vi "Find_Binary_Wavedump.vi"(8 "Time Limit (s)":u32) -> (12 "File Not Found":bool, 13 "File Not Found 5":bool, 14 "File Not Found 2":bool, 15 "File Not Found 6":bool, 16 "File Not Found 3":bool, 17 "File Not Found 7":bool, 18 "File Not Found 4":bool, 19 "File Not Found 8":bool, 20 "File Found":bool, 21 "File Found 2":bool, 22 "File Found 3":bool, 23 "File Found 4":bool, 24 "File Found 5":bool, 25 "File Found 6":bool, 26 "File Found 7":bool, 27 "File Found 8":bool)   [LabVIEW 2018]
panel:
  in  "Channel":string[](array[string])
  in  "Test":string(combo)
  out "File Found":bool[](array[boolean])
  out "File Not Found":bool[](array[boolean])
  out "File Path Out 8":path
  out "Time Looking for File (s) 8":u32=17125
  out "File Path Out 7":path
  out "Time Looking for File (s) 7":u32=17125
  out "File Path Out 6":path
  out "Time Looking for File (s) 6":u32=17125
  out "File Path Out 5":path
  out "Time Looking for File (s) 5":u32=17125
  out "File Path Out 4":path
  out "Time Looking for File (s) 4":u32=17125
  out "File Path Out 3":path
  out "Time Looking for File (s) 3":u32=17125
  out "File Path Out 2":path
  out "Time Looking for File (s) 2":u32=17125
  out "File Path Out":path
  out "Time Looking for File (s)":u32=17125
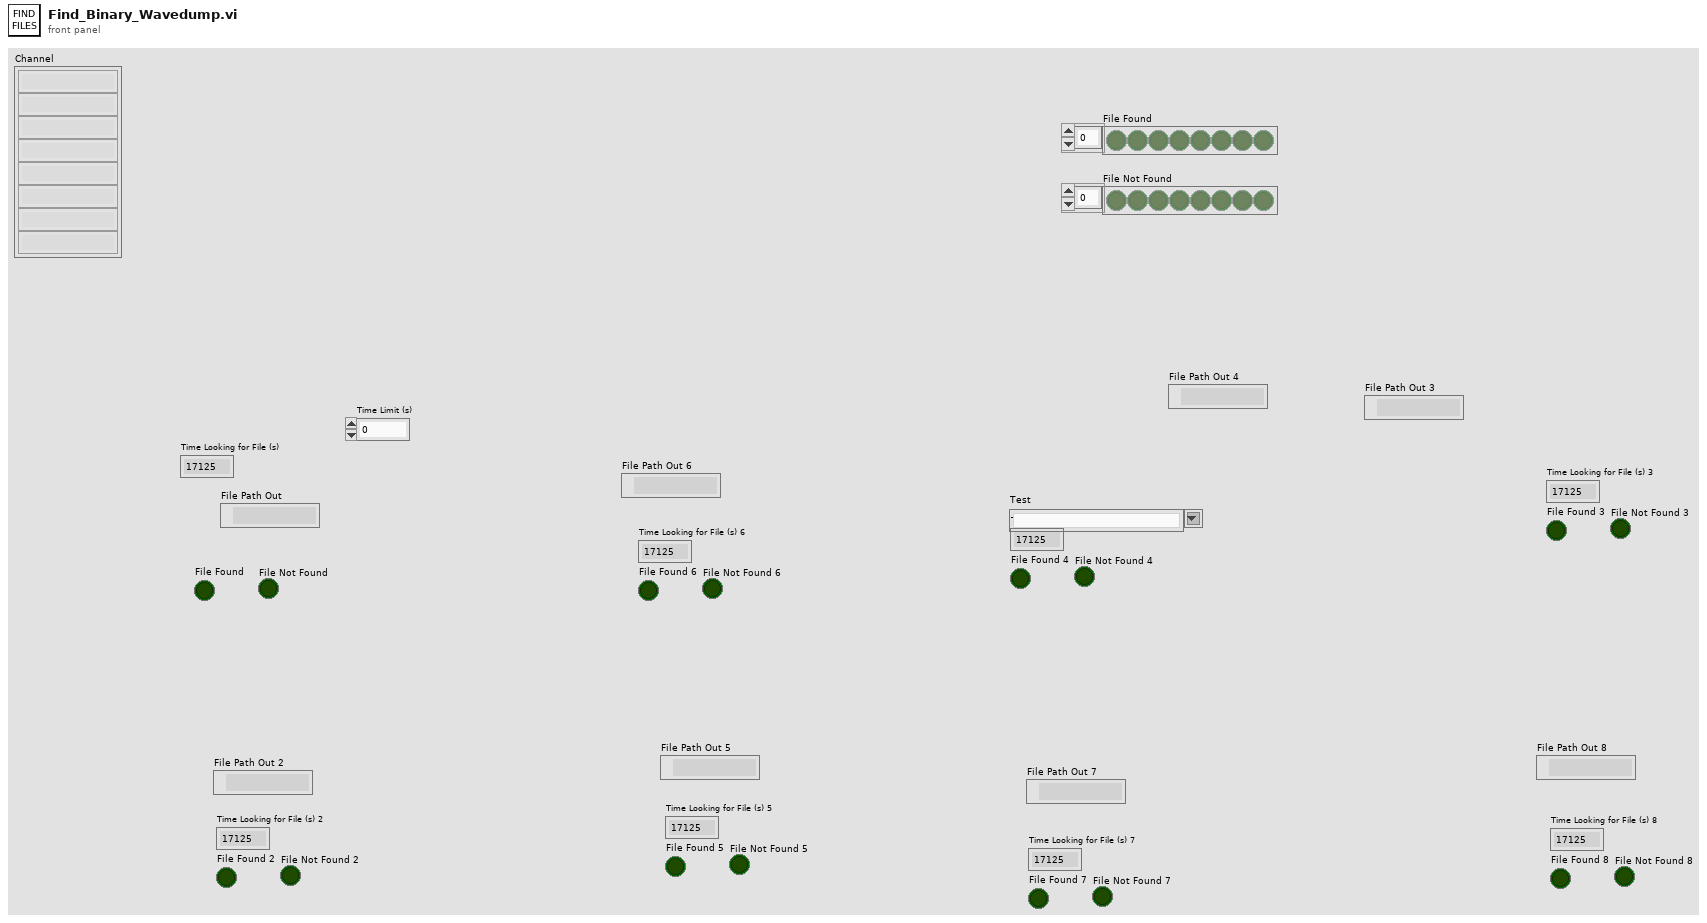
[diagram p1: front panel]
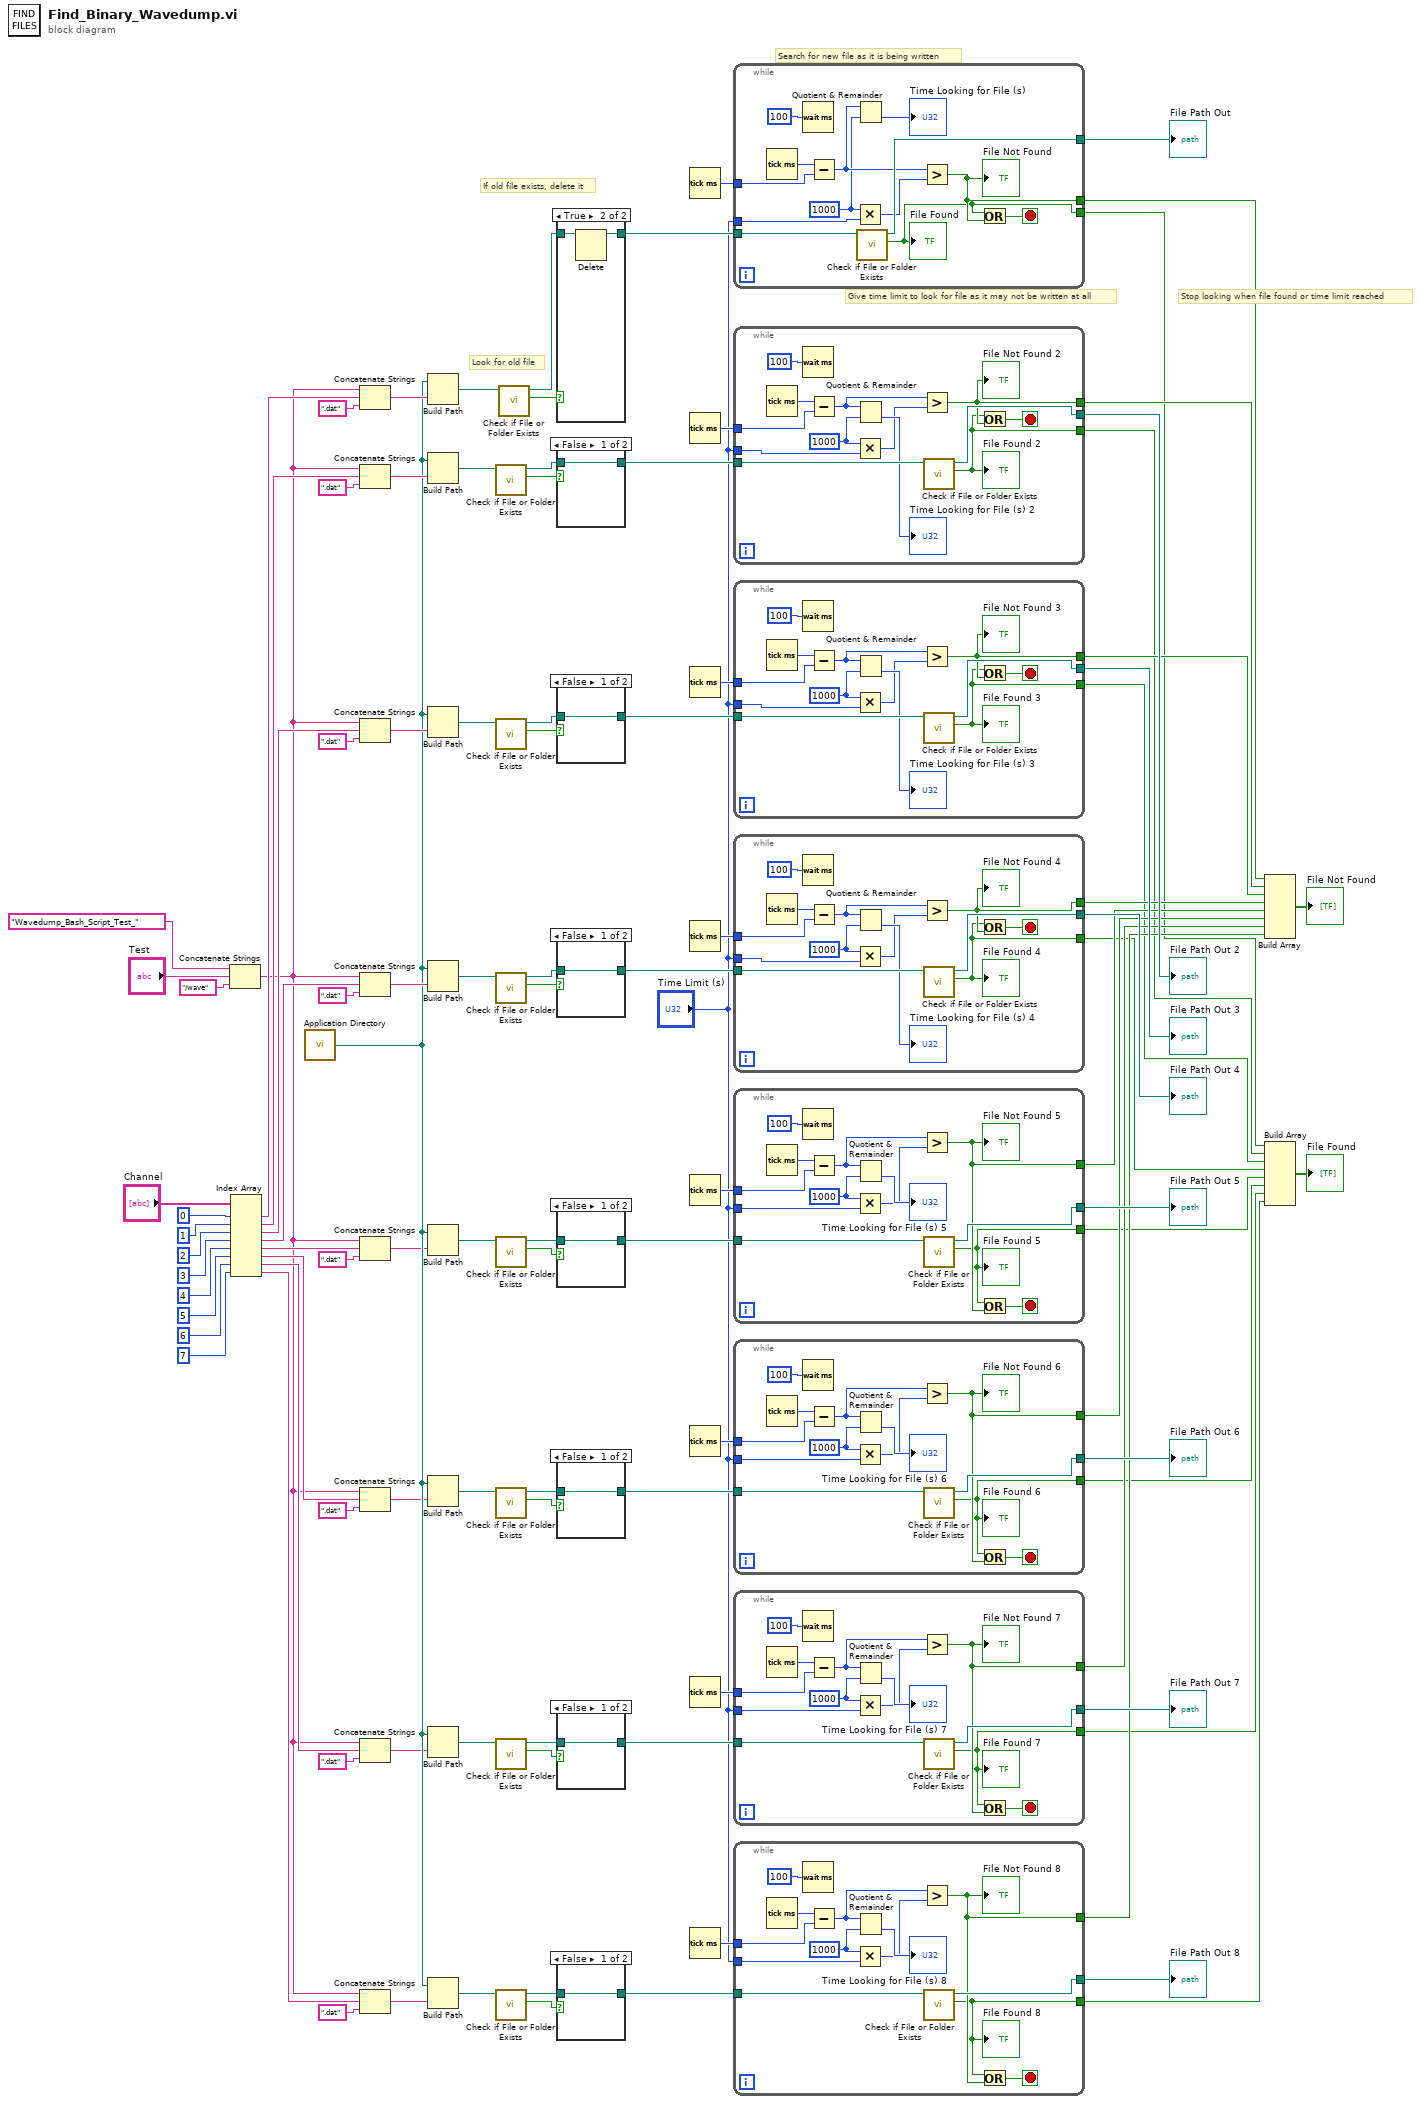
[diagram p0: block diagram]
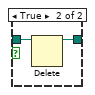
[diagram p2: hidden frame]
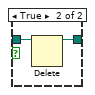
[diagram p3: hidden frame]
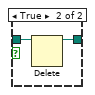
[diagram p4: hidden frame]
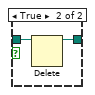
[diagram p5: hidden frame]
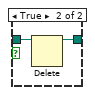
[diagram p6: hidden frame]
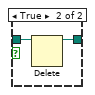
[diagram p7: hidden frame]
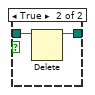
[diagram p8: hidden frame]
diagram:
  # "Stop looking when file found or time limit reached"
  # "Give time limit to look for file as it may not be written at all"
  # "Search for new file as it is being written"
  # "Look for old file"
  # "If old file exists, delete it"
  n1 = Concatenate Strings("Wavedump_Bash_Script_Test_" ("string"), "Test", "/wave" ("string")) -> (w16:string)
  n2 = Index Array(array="Channel", index #1=0 ("index"), index #2=1 ("index"), index #3=2 ("index"), index #4=3 ("index"), index #5=4 ("index"), index #6=5 ("index"), index #7=6 ("index"), index #8=7 ("index")) -> (element #1=w31:string, element #2=w23:string, element #3=w22:string, element #4=w21:string, element #5=w20:string, element #6=w19:string, element #7=w18:string, element #8=w17:string)
  n3 = call <vilib>:"Application Directory.vi"() -> ("Application Directory"=w11:path)
  n4 = Concatenate Strings(w16, w31, ".dat" ("string")) -> (w42:string)
  n5 = Concatenate Strings(w16, w23, ".dat" ("string")) -> (w14:string)
  n6 = Concatenate Strings(w16, w22, ".dat" ("string")) -> (w15:string)
  n7 = Concatenate Strings(w16, w21, ".dat" ("string")) -> (w13:string)
  n8 = Concatenate Strings(w16, w20, ".dat" ("string")) -> (w10:string)
  n9 = Concatenate Strings(w16, w19, ".dat" ("string")) -> (w9:string)
  n10 = Concatenate Strings(w16, w18, ".dat" ("string")) -> (w8:string)
  n11 = Concatenate Strings(w16, w17, ".dat" ("string")) -> (w7:string)
  n12 = Build Path(base path=w11, name or relative path=w42) -> (appended path=w30:path)
  n13 = Build Path(base path=w11, name or relative path=w14) -> (appended path=w12:path)
  n14 = Build Path(base path=w11, name or relative path=w15) -> (appended path=w6:path)
  n15 = Build Path(base path=w11, name or relative path=w13) -> (appended path=w5:path)
  n16 = Build Path(base path=w11, name or relative path=w10) -> (appended path=w4:path)
  n17 = Build Path(base path=w11, name or relative path=w9) -> (appended path=w1:path)
  n18 = Build Path(base path=w11, name or relative path=w8) -> (appended path=w3:path)
  n19 = Build Path(base path=w11, name or relative path=w7) -> (appended path=w2:path)
  n20 = call <vilib>:"Check if File or Folder Exists.vi"("path"=w12) -> ("file or folder exists?"=w99:bool, "dup path"=w100:path)  [unwired: 8 in, 1 out]
  n21 = call <vilib>:"Check if File or Folder Exists.vi"("path"=w6) -> ("file or folder exists?"=w94:bool, "dup path"=w95:path)  [unwired: 8 in, 1 out]
  n22 = call <vilib>:"Check if File or Folder Exists.vi"("path"=w5) -> ("file or folder exists?"=w89:bool, "dup path"=w90:path)  [unwired: 8 in, 1 out]
  n23 = call <vilib>:"Check if File or Folder Exists.vi"("path"=w4) -> ("file or folder exists?"=w84:bool, "dup path"=w85:path)  [unwired: 8 in, 1 out]
  n24 = call <vilib>:"Check if File or Folder Exists.vi"("path"=w1) -> ("file or folder exists?"=w79:bool, "dup path"=w80:path)  [unwired: 8 in, 1 out]
  n25 = call <vilib>:"Check if File or Folder Exists.vi"("path"=w3) -> ("file or folder exists?"=w74:bool, "dup path"=w75:path)  [unwired: 8 in, 1 out]
  n26 = call <vilib>:"Check if File or Folder Exists.vi"("path"=w2) -> ("file or folder exists?"=w69:bool, "dup path"=w70:path)  [unwired: 8 in, 1 out]
  n27 = call <vilib>:"Check if File or Folder Exists.vi"("path"=w30) -> ("file or folder exists?"=w104:bool, "dup path"=w105:path)  [unwired: 8 in, 1 out]
  n28 = case shown="True" w104 {
    tunnel: w105 -> [w106 w108]
    tunnel: [w106 w107] -> w103
    frame False {
    }
    frame True {
      n29 = Delete(path (use dialog)=w108) -> (deleted path=w107:path)  [unwired: 4 in, 2 out]
    }
  }
  n30 = case shown="False" w99 {
    tunnel: w100 -> [w109 w111]
    tunnel: [w109 w110] -> w98
    frame False {
    }
    frame True {
      n31 = Delete(path (use dialog)=w111) -> (deleted path=w110:path)  [unwired: 4 in, 2 out]
    }
  }
  n32 = case shown="False" w94 {
    tunnel: w95 -> [w112 w114]
    tunnel: [w112 w113] -> w93
    frame False {
    }
    frame True {
      n33 = Delete(path (use dialog)=w114) -> (deleted path=w113:path)  [unwired: 4 in, 2 out]
    }
  }
  n34 = case shown="False" w89 {
    tunnel: w90 -> [w115 w117]
    tunnel: [w115 w116] -> w88
    frame False {
    }
    frame True {
      n35 = Delete(path (use dialog)=w117) -> (deleted path=w116:path)  [unwired: 4 in, 2 out]
    }
  }
  n36 = case shown="False" w84 {
    tunnel: w85 -> [w118 w120]
    tunnel: [w118 w119] -> w83
    frame False {
    }
    frame True {
      n37 = Delete(path (use dialog)=w120) -> (deleted path=w119:path)  [unwired: 4 in, 2 out]
    }
  }
  n38 = case shown="False" w79 {
    tunnel: w80 -> [w121 w123]
    tunnel: [w121 w122] -> w78
    frame False {
    }
    frame True {
      n39 = Delete(path (use dialog)=w123) -> (deleted path=w122:path)  [unwired: 4 in, 2 out]
    }
  }
  n40 = case shown="False" w74 {
    tunnel: w75 -> [w124 w126]
    tunnel: [w124 w125] -> w73
    frame False {
    }
    frame True {
      n41 = Delete(path (use dialog)=w126) -> (deleted path=w125:path)  [unwired: 4 in, 2 out]
    }
  }
  n42 = case shown="False" w69 {
    tunnel: w70 -> [w127 w129]
    tunnel: [w127 w128] -> w68
    frame False {
    }
    frame True {
      n43 = Delete(path (use dialog)=w129) -> (deleted path=w128:path)  [unwired: 4 in, 2 out]
    }
  }
  n44 = Tick Count (ms)() -> (millisecond timer value=w102:u32)
  n45 = Tick Count (ms)() -> (millisecond timer value=w97:u32)
  n46 = Tick Count (ms)() -> (millisecond timer value=w92:u32)
  n47 = Tick Count (ms)() -> (millisecond timer value=w87:u32)
  n48 = Tick Count (ms)() -> (millisecond timer value=w82:u32)
  n49 = Tick Count (ms)() -> (millisecond timer value=w77:u32)
  n50 = Tick Count (ms)() -> (millisecond timer value=w72:u32)
  n51 = Tick Count (ms)() -> (millisecond timer value=w67:u32)
  n52 = while {
    tunnel: [w142] -> w101
    tunnel: w102 -> [w140]
    tunnel: w103 -> [w138]
    tunnel: [w136] -> w65
    tunnel: "Time Limit (s)" -> [w131]
    tunnel: [w130] -> w48
    stop <- w137 stop-if-true
    w133 = u32 1000 ("y")
    n53 = Tick Count (ms)() -> (millisecond timer value=w139:u32)
    n54 = Wait (ms)(milliseconds to wait=100) -> ()  [unwired: 1 out]
    n55 = Subtract(x=w139, y=w140) -> (x-y=w134:u32)
    n56 = Multiply(x=w133, y=w131) -> (x*y=w132:u32)
    n57 = Quotient & Remainder(x=w134, y=w133) -> (floor(x/y)=→"Time Looking for File (s)":u32)  [unwired: 1 out]
    n58 = call <vilib>:"Check if File or Folder Exists.vi"("path"=w138) -> ("file or folder exists?"=w130:bool, "dup path"=w142:path)  [unwired: 8 in, 1 out]
    "File Found" <- w130
    n59 = Greater?(x=w134, y=w132) -> (0:w136:bool)
    "File Not Found" <- w136
    n60 = Or(x=w130, y=w136) -> (x .or. y?=w137:bool)
  }
  "File Path Out" <- w101
  n61 = while {
    tunnel: [w155] -> w96
    tunnel: w97 -> [w153]
    tunnel: w98 -> [w151]
    tunnel: [w149] -> w64
    tunnel: "Time Limit (s)" -> [w144]
    tunnel: [w143] -> w50
    stop <- w150 stop-if-true
    w146 = u32 1000 ("y")
    n62 = Tick Count (ms)() -> (millisecond timer value=w152:u32)
    n63 = Wait (ms)(milliseconds to wait=100) -> ()  [unwired: 1 out]
    n64 = Subtract(x=w152, y=w153) -> (x-y=w147:u32)
    n65 = Multiply(x=w146, y=w144) -> (x*y=w145:u32)
    n66 = Quotient & Remainder(x=w147, y=w146) -> (floor(x/y)=→"Time Looking for File (s) 2":u32)  [unwired: 1 out]
    n67 = Greater?(x=w147, y=w145) -> (0:w149:bool)
    "File Not Found 2" <- w149
    n68 = call <vilib>:"Check if File or Folder Exists.vi"("path"=w151) -> ("file or folder exists?"=w143:bool, "dup path"=w155:path)  [unwired: 8 in, 1 out]
    "File Found 2" <- w143
    n69 = Or(x=w143, y=w149) -> (x .or. y?=w150:bool)
  }
  "File Path Out 2" <- w96
  n70 = while {
    tunnel: [w168] -> w91
    tunnel: w92 -> [w166]
    tunnel: w93 -> [w164]
    tunnel: [w162] -> w63
    tunnel: "Time Limit (s)" -> [w157]
    tunnel: [w156] -> w49
    stop <- w163 stop-if-true
    w159 = u32 1000 ("y")
    n71 = Tick Count (ms)() -> (millisecond timer value=w165:u32)
    n72 = Wait (ms)(milliseconds to wait=100) -> ()  [unwired: 1 out]
    n73 = Subtract(x=w165, y=w166) -> (x-y=w160:u32)
    n74 = Multiply(x=w159, y=w157) -> (x*y=w158:u32)
    n75 = Quotient & Remainder(x=w160, y=w159) -> (floor(x/y)=→"Time Looking for File (s) 3":u32)  [unwired: 1 out]
    n76 = Greater?(x=w160, y=w158) -> (0:w162:bool)
    "File Not Found 3" <- w162
    n77 = call <vilib>:"Check if File or Folder Exists.vi"("path"=w164) -> ("file or folder exists?"=w156:bool, "dup path"=w168:path)  [unwired: 8 in, 1 out]
    "File Found 3" <- w156
    n78 = Or(x=w156, y=w162) -> (x .or. y?=w163:bool)
  }
  "File Path Out 3" <- w91
  n79 = while {
    tunnel: [w181] -> w86
    tunnel: w87 -> [w179]
    tunnel: w88 -> [w177]
    tunnel: [w175] -> w62
    tunnel: "Time Limit (s)" -> [w170]
    tunnel: [w169] -> w51
    stop <- w176 stop-if-true
    w172 = u32 1000 ("y")
    n80 = Tick Count (ms)() -> (millisecond timer value=w178:u32)
    n81 = Wait (ms)(milliseconds to wait=100) -> ()  [unwired: 1 out]
    n82 = Subtract(x=w178, y=w179) -> (x-y=w173:u32)
    n83 = Multiply(x=w172, y=w170) -> (x*y=w171:u32)
    n84 = Quotient & Remainder(x=w173, y=w172) -> (floor(x/y)=→"Time Looking for File (s) 4":u32)  [unwired: 1 out]
    n85 = Greater?(x=w173, y=w171) -> (0:w175:bool)
    "File Not Found 4" <- w175
    n86 = call <vilib>:"Check if File or Folder Exists.vi"("path"=w177) -> ("file or folder exists?"=w169:bool, "dup path"=w181:path)  [unwired: 8 in, 1 out]
    "File Found 4" <- w169
    n87 = Or(x=w169, y=w175) -> (x .or. y?=w176:bool)
  }
  "File Path Out 4" <- w86
  n88 = while {
    tunnel: [w194] -> w81
    tunnel: w82 -> [w192]
    tunnel: w83 -> [w190]
    tunnel: [w188] -> w61
    tunnel: "Time Limit (s)" -> [w183]
    tunnel: [w182] -> w52
    stop <- w189 stop-if-true
    w185 = u32 1000 ("y")
    n89 = Tick Count (ms)() -> (millisecond timer value=w191:u32)
    n90 = Wait (ms)(milliseconds to wait=100) -> ()  [unwired: 1 out]
    n91 = Subtract(x=w191, y=w192) -> (x-y=w186:u32)
    n92 = Multiply(x=w185, y=w183) -> (x*y=w184:u32)
    n93 = Quotient & Remainder(x=w186, y=w185) -> (floor(x/y)=→"Time Looking for File (s) 5":u32)  [unwired: 1 out]
    n94 = Greater?(x=w186, y=w184) -> (0:w188:bool)
    "File Not Found 5" <- w188
    n95 = call <vilib>:"Check if File or Folder Exists.vi"("path"=w190) -> ("file or folder exists?"=w182:bool, "dup path"=w194:path)  [unwired: 8 in, 1 out]
    "File Found 5" <- w182
    n96 = Or(x=w182, y=w188) -> (x .or. y?=w189:bool)
  }
  "File Path Out 5" <- w81
  n97 = while {
    tunnel: [w207] -> w76
    tunnel: w77 -> [w205]
    tunnel: w78 -> [w203]
    tunnel: [w201] -> w60
    tunnel: "Time Limit (s)" -> [w196]
    tunnel: [w195] -> w53
    stop <- w202 stop-if-true
    w198 = u32 1000 ("y")
    n98 = Tick Count (ms)() -> (millisecond timer value=w204:u32)
    n99 = Wait (ms)(milliseconds to wait=100) -> ()  [unwired: 1 out]
    n100 = Subtract(x=w204, y=w205) -> (x-y=w199:u32)
    n101 = Multiply(x=w198, y=w196) -> (x*y=w197:u32)
    n102 = Quotient & Remainder(x=w199, y=w198) -> (floor(x/y)=→"Time Looking for File (s) 6":u32)  [unwired: 1 out]
    n103 = Greater?(x=w199, y=w197) -> (0:w201:bool)
    "File Not Found 6" <- w201
    n104 = call <vilib>:"Check if File or Folder Exists.vi"("path"=w203) -> ("file or folder exists?"=w195:bool, "dup path"=w207:path)  [unwired: 8 in, 1 out]
    "File Found 6" <- w195
    n105 = Or(x=w195, y=w201) -> (x .or. y?=w202:bool)
  }
  "File Path Out 6" <- w76
  n106 = while {
    tunnel: [w220] -> w71
    tunnel: w72 -> [w218]
    tunnel: w73 -> [w216]
    tunnel: [w214] -> w59
    tunnel: "Time Limit (s)" -> [w209]
    tunnel: [w208] -> w54
    stop <- w215 stop-if-true
    w211 = u32 1000 ("y")
    n107 = Tick Count (ms)() -> (millisecond timer value=w217:u32)
    n108 = Wait (ms)(milliseconds to wait=100) -> ()  [unwired: 1 out]
    n109 = Subtract(x=w217, y=w218) -> (x-y=w212:u32)
    n110 = Multiply(x=w211, y=w209) -> (x*y=w210:u32)
    n111 = Quotient & Remainder(x=w212, y=w211) -> (floor(x/y)=→"Time Looking for File (s) 7":u32)  [unwired: 1 out]
    n112 = Greater?(x=w212, y=w210) -> (0:w214:bool)
    "File Not Found 7" <- w214
    n113 = call <vilib>:"Check if File or Folder Exists.vi"("path"=w216) -> ("file or folder exists?"=w208:bool, "dup path"=w220:path)  [unwired: 8 in, 1 out]
    "File Found 7" <- w208
    n114 = Or(x=w208, y=w214) -> (x .or. y?=w215:bool)
  }
  "File Path Out 7" <- w71
  n115 = while {
    tunnel: [w233] -> w66
    tunnel: w67 -> [w231]
    tunnel: w68 -> [w229]
    tunnel: [w227] -> w58
    tunnel: "Time Limit (s)" -> [w222]
    tunnel: [w221] -> w55
    stop <- w228 stop-if-true
    w224 = u32 1000 ("y")
    n116 = Tick Count (ms)() -> (millisecond timer value=w230:u32)
    n117 = Wait (ms)(milliseconds to wait=100) -> ()  [unwired: 1 out]
    n118 = Subtract(x=w230, y=w231) -> (x-y=w225:u32)
    n119 = Multiply(x=w224, y=w222) -> (x*y=w223:u32)
    n120 = Quotient & Remainder(x=w225, y=w224) -> (floor(x/y)=→"Time Looking for File (s) 8":u32)  [unwired: 1 out]
    n121 = Greater?(x=w225, y=w223) -> (0:w227:bool)
    "File Not Found 8" <- w227
    n122 = call <vilib>:"Check if File or Folder Exists.vi"("path"=w229) -> ("file or folder exists?"=w221:bool, "dup path"=w233:path)  [unwired: 8 in, 1 out]
    "File Found 8" <- w221
    n123 = Or(x=w221, y=w227) -> (x .or. y?=w228:bool)
  }
  "File Path Out 8" <- w66
  n124 = Build Array(w65, w64, w63, w62, w61, w60, w59, w58) -> (→"File Not Found":bool[])
  n125 = Build Array(w48, w50, w49, w51, w52, w53, w54, w55) -> (→"File Found":bool[])
